vi "vis_acq_disassemble_finiteInline.vi"(4 "Number of Images":i32=10, 7 "error in":errorcluster) -> (20 "Image Out":T2(plugin-control), 21 "All Images Out":T2[](array[typedef]), 26 "Stopped":bool, 27 "error out":errorcluster)   [LabVIEW 2013]
doc: "Creates, and edits acquisitions using the NI Vision Acquisition Express VI.\n\nThe NI Vision Acquisition Wizard is launched by placing the Express VI on the block diagram. Select an acquisition source and configure an acquisition using NI-IMAQ, NI-IMAQdx, or simulate an acquisition by reading an AVI or image files from a folder. After an acquisition is configured, select controls and indicators to be able to programmatically set in LabVIEW. Double-click the Vision Acquisition Express VI to edit the acquisition.\n\nNote: Any images created by the Express VI need to be disposed after use. Use the IMAQ Dispose.vi to cleanup the images output by the Express VI when they are no longer needed."
uses:
  <vilib>/vision/Image Controls.llb/IMAQ Image.ctl
  <vilib>/userdefined/High Color/IMAQdx.ctl
  <vilib>/vision/driver/NI_Vision_Acquisition_Software.lvlib
panel:
  out "Session Out":T1
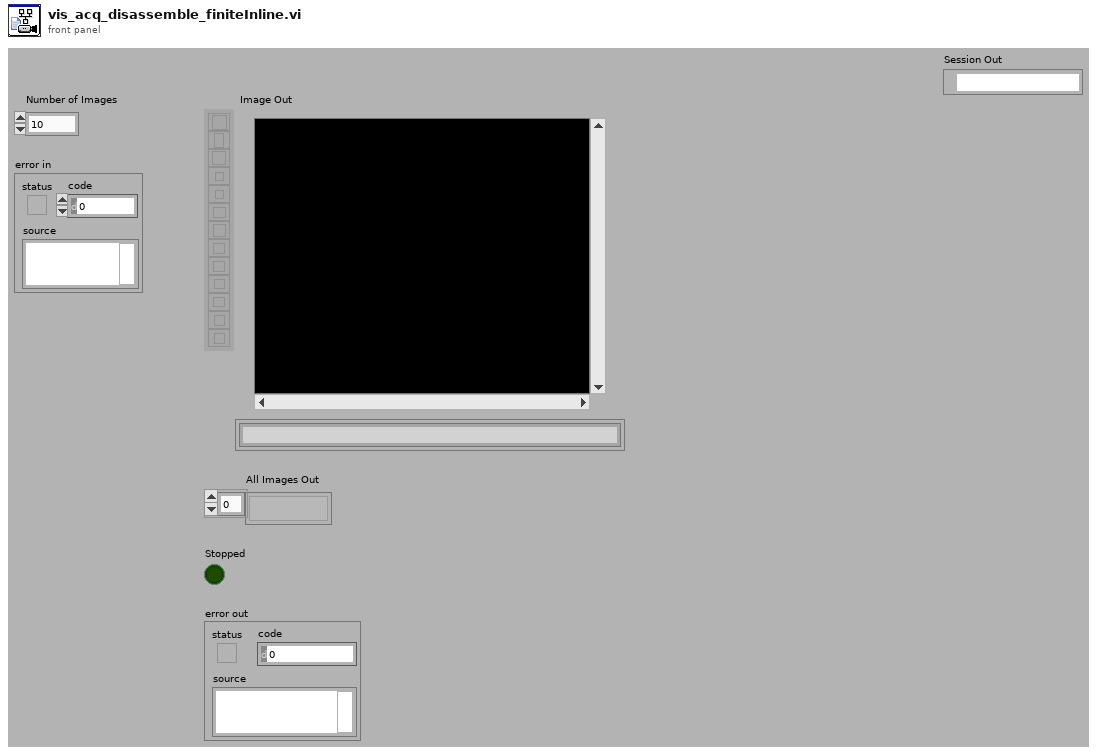
[diagram p1: front panel]
types:
  T1 = typedef "IMAQdx.ctl" = refnum<k21>
  T2 = typedef "IMAQ Image.ctl" = refnum<image>
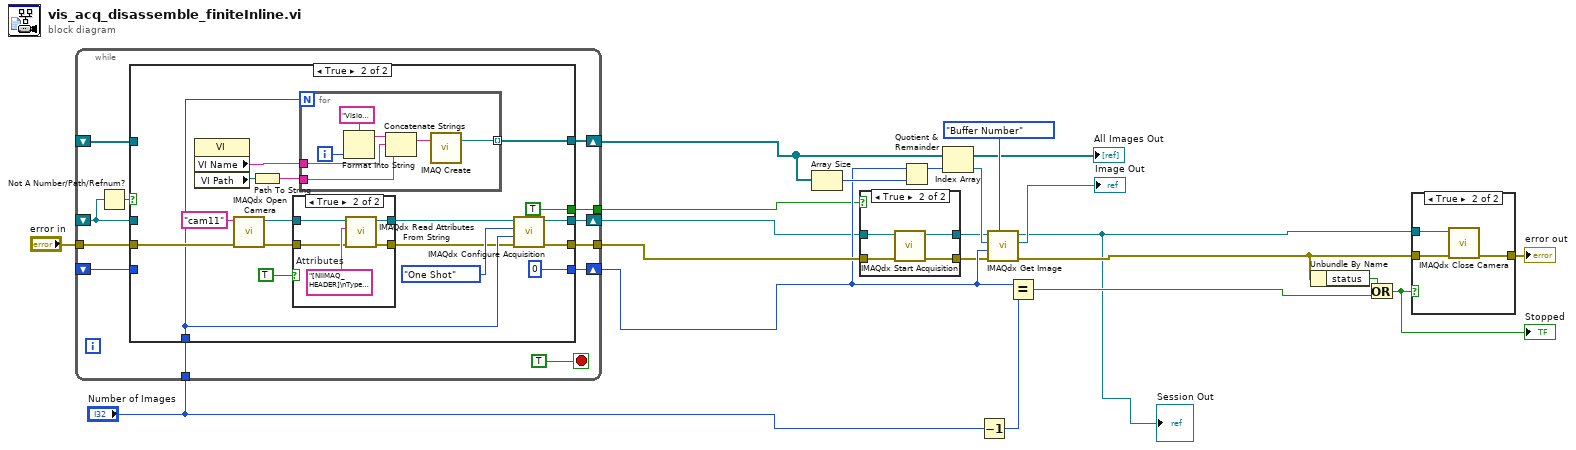
[diagram p0: block diagram]
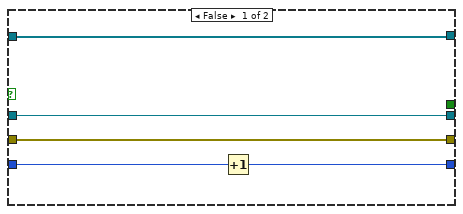
[diagram p4: hidden frame]
diagram:
  n1 = while {
    shift-right: [w33] -> w9
    shift-left: _ -> [w24]
    tunnel: [w32] -> w20
    tunnel: "error in" -> [w31]
    shift-right: [w29] -> w13
    shift-left: _ -> [w28]
    shift-right: [w27] -> w10
    shift-left: _ -> [w26]
    tunnel: "Number of Images" -> [w25]
    tunnel: [w22] -> w6
    stop <- TRUE stop-if-true
    n2 = Not A Number/Path/Refnum?(number/path/refnum=w24) -> (NaN/Path/Refnum?=w23:bool)
    n3 = case shown="True" w23 {
      tunnel: [w38 w52] -> w33
      tunnel: w24 -> [w38 _]
      tunnel: [w37 w51] -> w32
      tunnel: w31 -> [w37 w55]
      tunnel: [w36 w53] -> w29
      tunnel: w28 -> [w36 _]
      tunnel: [w34 0] -> w27
      tunnel: w26 -> [w35 _]
      tunnel: w25 -> [_ w48]
      tunnel: [_ TRUE] -> w22
      frame False {
        n4 = Increment(x=w35) -> (x+1=w34:i32)
      }
      frame True {
        n5 = property class="VI"() -> ("VI Name"=w46:string, "VI Path"=w47:path)  [unwired: 2 in, 2 out]
        n6 = call <vilib>:"IMAQdx Open Camera.vi"("error in"=w55, "Session In"="cam11" ("Interface Name")) -> ("error out"=w43:errorcluster, "Session Out"=w44:T1)  [unwired: 1 in, 7 out]
        n7 = Path To String(path=w47) -> (string=w45:string)
        n8 = case shown="True" TRUE ("Init Attributes") {
          tunnel: w44 -> [w57 w62]
          tunnel: w43 -> [w56 w60]
          tunnel: [w57 w59] -> w42
          tunnel: [w56 w58] -> w41
          frame False {
          }
          frame True {
            w61 = "[NIIMAQ_HEADER]\nType = 2\nVersion = 8\n\n[CAMERA_DATA]\nAcquisitionAttributes::Bayer::Algorithm = \"Bilinear\"\nAcquisitionAttributes::Bayer::GainB = \"1\"\nAcquisitionAttributes::Bayer::GainG = \"1\"\nAcquisitionAttributes::Bayer::GainR = \"1\"\nAcquisitionAttributes::Bayer::Pattern = \"Use hardware value\"\nAcquisitionAttributes::BitsPerPixel = \"Use hardware value\"\nAcquisitionAttributes::IgnoreFirstFrame = \"false\"\nAcquisitionAttributes::ImageDecoderCopyMode = \"Auto\"\nAcquisitionAttributes::OutputImageType = \"Auto\"\nAcquisitionAttributes::OverwriteMode = \"Get Newest\"\nAcquisitionAttributes::PixelSignedness = \"Use hardware value\"\nAcquisitionAttributes::ReceiveTimestampMode = \"None\"\nAcquisitionAttributes::ShiftPixelBits = \"false\"\nAcquisitionAttributes::SwapPixelBytes = \"false\"\nAcquisitionAttributes::Timeout = \"5000\"\nAcquisitionAttributes::VerticalMirror = \"false\"\nAcquisitionAttributes::VideoMode = \"1280x720 RGB24 30.00fps\"\nCameraAttributes::BacklightCompensation::Mode = \"Manual\"\nCameraAttributes::BacklightCompensation::Value = \"false\"\nCameraAttributes::Brightness::Mode = \"Manual\"\nCameraAttributes::Brightness::Value = \"133\"\nCameraAttributes::Contrast::Mode = \"Manual\"\nCameraAttributes::Contrast::Value = \"0.050000000000000003\"\nCameraAttributes::Exposure::Mode = \"Auto\"\nCameraAttributes::Pan::Mode = \"Manual\"\nCameraAttributes::Pan::Value = \"0\"\nCameraAttributes::Saturation::Mode = \"Manual\"\nCameraAttributes::Saturation::Value = \"83\"\nCameraAttributes::Sharpness::Mode = \"Manual\"\nCameraAttributes::Sharpness::Value = \"25\"\nCameraAttributes::Tilt::Mode = \"Manual\"\nCameraAttributes::Tilt::Value = \"0\"\nCameraAttributes::WhiteBalance::Mode = \"Auto\"\nCameraAttributes::Zoom::Mode = \"Manual\"\nCameraAttributes::Zoom::Value = \"0\"\n"  # Attributes
            n9 = call <vilib>:"IMAQdx Read Attributes From String.vi"("error in"=w60, "Attributes String In"=w61, "Session In"=w62) -> ("error out"=w58:errorcluster, "Session Out"=w59:T1)  [unwired: 7 out]
          }
        }
        n10 = for {
          N: w48 -> [_]
          tunnel: [w69] -> w53 mode=indexing
          tunnel: w46 -> [w64]
          tunnel: w45 -> [w63]
          i -> [w68]
          n11 = Format Into String(format string="Vision Acq Image 193232353 %d" ("Image Name"), w68) -> (resulting string=w66:string)  [unwired: 2 in, 1 out]
          n12 = Concatenate Strings(w66, w64, w63) -> (w65:string)
          n13 = call "IMAQ Create"("Image Name"=w65) -> ("New Image"=w69:T2)  [unwired: 3 in, 2 out]
        }
        n14 = call <vilib>:"IMAQdx Configure Acquisition.vi"("error in"=w41, "Number of Buffers"=w48, "Continuous?"=enum32{"One Shot", "Continuous"}."One Shot" ("Mode"), "Session In"=w42) -> ("error out"=w51:errorcluster, "Session Out"=w52:T1)  [unwired: 6 out]
      }
    }
  }
  "All Images Out" <- w13
  n15 = Array Size(array=w13) -> (size(s)=w15:i32)
  n16 = case shown="True" w6 {
    tunnel: w9 -> [w71 w75]
    tunnel: w20 -> [w70 w74]
    tunnel: [w70 w73] -> w7
    tunnel: [w71 w72] -> w8
    frame False {
    }
    frame True {
      n17 = call <vilib>:"IMAQdx Start Acquisition.vi"("error in"=w74, "Session In"=w75) -> ("error out"=w73:errorcluster, "Session Out"=w72:T1)  [unwired: 8 out]
    }
  }
  n18 = Quotient & Remainder(x=w10, y=w15) -> (x-y*floor(x/y)=w14:i32)  [unwired: 1 out]
  n19 = Index Array(array=w13, index=w14) -> (element=w12:T2)
  n20 = Decrement(x="Number of Images") -> (x-1=w17:i32)
  n21 = call <vilib>:"IMAQdx Get Image.vi"("Buffer Number Mode (Next)"=enum32{"Next", "Last", "Buffer Number"}."Buffer Number", "error in"=w7, "Buffer Number In"=w10, "Image In"=w12, "Session In"=w8) -> ("error out"=w11:errorcluster, "Image Out"=→"Image Out":T2, "Session Out"=w1:T1)  [unwired: 4 out]
  "Session Out" <- w1
  n22 = Equal?(x=w10, y=w17) -> (x = y?=w4:bool)
  n23 = Unbundle By Name(w11) -> ("status"=w2:bool)
  n24 = Or(x=w2, y=w4) -> (x .or. y?=w3:bool)
  "Stopped" <- w3
  n25 = case "Case Structure_template1" shown="True" w3 {
    tunnel: [w76 w78] -> w5
    tunnel: w11 -> [w76 w79]
    tunnel: w1 -> [_ w77]
    frame False {
    }
    frame True {
      n26 = call <vilib>:"IMAQdx Close Camera.vi"("error in"=w79, "Session In"=w77) -> ("error out"=w78:errorcluster)  [unwired: 9 out]
    }
  }
  "error out" <- w5
